vi "2 Steering Chooser.vi"() -> (2 "rudder setpoint":T1=-30.0 format="%05.1f")   [LabVIEW 2011]
doc: "Takes waypoint and boat location information from the global variable and places the approproate rudder position command on the global.\nFor Drive waypoints, this VI simply tries to make the boat's heading the same as the heading between the boat and the waypoint. TODO: this does not account for drift -- it assumes that the boat will go where it is pointed which is not always the case.\n\nTODO: important: As of 11/17 this VI only works for the Drive option.\nTODO: ideally this VI would run on any update of the boat location or waypoint location, and not otherwise."
uses:
  2 Typedefs/heading.ctl
  0x2-OCU-Think Comm/0x2 Typedefs/ocuWaypoint.ctl
  0x2-OCU-Think Comm/0x2 Typedefs/waypointTypes.ctl
  2 Typedefs/UTM Location.ctl
  2 Typedefs/Velocity.ctl
  2 Globals/2 Global.vi
panel:
  in  "maximum rudder deflection":T1=-30.0 format="%05.1f"
  out "Robot\nHeading":T1 format="%05.1f"
  out "Angle to waypt":T1 format="%05.1f"
  out "Distance to Waypoint":T2
  out "Robot UTM Location":T3 {"North" format="%#_10f"; "East" format="%#_8f"}
  out "Waypoint":T4 {"UTM Location"."North" format="%#_10f"; "UTM Location"."East" format="%#_8f"}
  out "desired delta heading":T1 format="%05.1f"
  # "Steering Chooser simply turns the rudder to aim the boat's bow towards the next waypoint.\n\nTODO: currently only implements Drive waypoints. Also this is extremely stupid.\nImplement avoidance, stay-in-area, and maybe a PID loop."
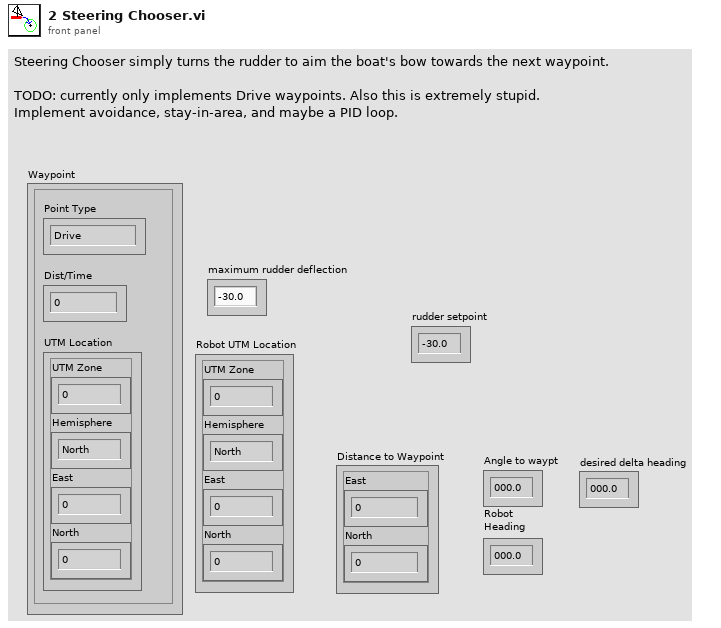
[diagram p1: front panel]
types:
  T1 = typedef "heading.ctl" = dbl
  T2 = typedef "Velocity.ctl" = cluster{"East":dbl, "North":dbl}
  T3 = typedef "UTM Location.ctl" = cluster{"UTM Zone":dbl, "Hemisphere":enum16{"North", "South"}, "East":dbl, "North":dbl}
  T4 = typedef "ocuWaypoint.ctl" = cluster{"Point Type":T5, "Dist/Time":dbl, "UTM Location":T3}
  T5 = typedef "waypointTypes.ctl" = enum16{"Drive", "Round Port", "Round Starboard", "Stay"}
  T6 = typedef "Current Waypoint.ctl" = i32
  T7 = typedef "Waypoints List.ctl" = T4[]
  T8 = cluster{"UTM Zone":dbl, "Hemisphere":u16, "East":dbl, "North":dbl}
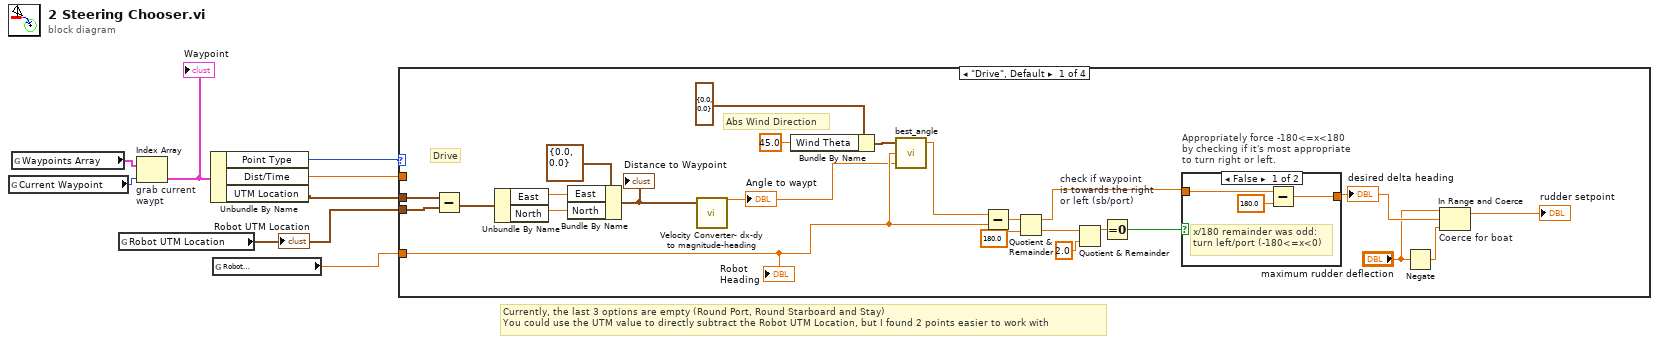
[diagram p0: block diagram]
diagram:
  # "Currently, the last 3 options are empty (Round Port, Round Starboard and Stay)\nYou could use the UTM value to directly subtract the Robot UTM Location, but I found 2 points easier to work with"
  n1 = global read "2 Global.vi" "Current Waypoint"() -> (w1:T6)
  n2 = global read "2 Global.vi" "Waypoints Array"() -> (w2:T7)
  n3 = global read "2 Global.vi" "Robot UTM Location"() -> (w8:T3)
  "Robot UTM Location" <- w8
  n4 = Index Array "grab current\nwaypt"(array=w2, index=w1) -> (element=w6:T4)
  "Waypoint" <- w6
  n5 = Unbundle By Name(w6) -> ("Point Type"=w3:T5, "Dist/Time"=w4:dbl, "UTM Location"=w5:T3)
  n6 = global read "2 Global.vi" "Robot\nHeading"() -> (w7:T1)
  n7 = case shown="\"Drive\", Default" w3 {
    tunnel: w5 -> [w32 _ _ _]
    tunnel: w8 -> [w31 _ _ _]
    tunnel: w7 -> [w11 _ _ _]
    tunnel: w4 -> [_ _ _ _]
    frame "Drive", Default {
      # "Abs Wind Direction"
      # "Drive"
      n8 = Subtract(x=w32, y=w31) -> (x-y=w30:T8)
      n9 = Unbundle By Name(w30) -> ("East"=w29:dbl, "North"=w28:dbl)
      n10 = Bundle By Name(cluster=T2 {"East"=0.0, "North"=0.0} ("Vector In"), "East"=w29, "North"=w28) -> (w26:T2)
      "Distance to Waypoint" <- w26
      n11 = call "Velocity Converter- dx-dy to magnitude-heading.vi"("Vector In"=w26) -> ("Heading Out"=w10:T1)  [unwired: 9 in, 1 out]
      "Angle to waypt" <- w10
      n12 = Bundle By Name(cluster=cluster{"Wind R":dbl, "Wind Theta":dbl} {"Wind R"=0.0, "Wind Theta"=0.0} ("Wind Vector"), "Wind Theta"=45.0) -> (w14:cluster{"Wind R":dbl, "Wind Theta":dbl})
      n13 = call "best_angle.vi"("Waypoint Heading"=w10, "Current Heading"=w11, "Wind Vector"=w14) -> ("Best Angle"=w9:dbl)  [unwired: 2 out]
      n14 = Subtract(x=w9, y=w11) -> (x-y=w24:T1)
      n15 = Quotient & Remainder ("shift to -180<x<180")(x=w24, y=T1 180.0) -> (x-y*floor(x/y)=w19:T1, floor(x/y)=w23:T1)
      n16 = Quotient & Remainder ("shift to -180<x<180")(x=w23, y=T1 2.0) -> (x-y*floor(x/y)=w21:T1)  [unwired: 1 out]
      n17 = Equal To 0? "check if waypoint\nis towards the right\nor left (sb/port)"(x=w21) -> (x = 0?=w20:bool)
      n18 = case "Appropriately force -180<=x<180\nby checking if it's most appropriate\nto turn right or left." shown="False" w20 {
        tunnel: w19 -> [w34 w36]
        tunnel: [w33 w36] -> w18
        frame False {
          # "x/180 remainder was odd:\nturn left/port (-180<=x<0)"
          n19 = Subtract(x=w34, y=T1 180.0) -> (x-y=w33:T1)
        }
        frame True {
          # "x/180 remainder was\neven: turn right/sb\n(0<=x<180)"
        }
      }
      "desired delta heading" <- w18
      n20 = Negate(x="maximum rudder deflection") -> (-x=w16:T1)
      n21 = In Range and Coerce "Coerce for boat"(upper limit="maximum rudder deflection", x=w18, lower limit=w16) -> (coerced(x)=→"rudder setpoint":T1)  [unwired: 1 out]
      "Robot\nHeading" <- w11
    }
    frame "Round Port" {
      # "Round Port"
    }
    frame "Round Starboard" {
      # "Round Starboard"
    }
    frame "Stay" {
      # "Stay"
    }
  }
